vi "Read Perimeter.vi"(8 "error in (no error)":errorcluster, 11 "Circle in":refnum<class "Circle.lvclass">) -> (0 "error out":errorcluster, 2 "Perimeter":dbl, 3 "Circle out":refnum<class "Circle.lvclass">)   [LabVIEW 2015]
uses:
  Circle.lvclass
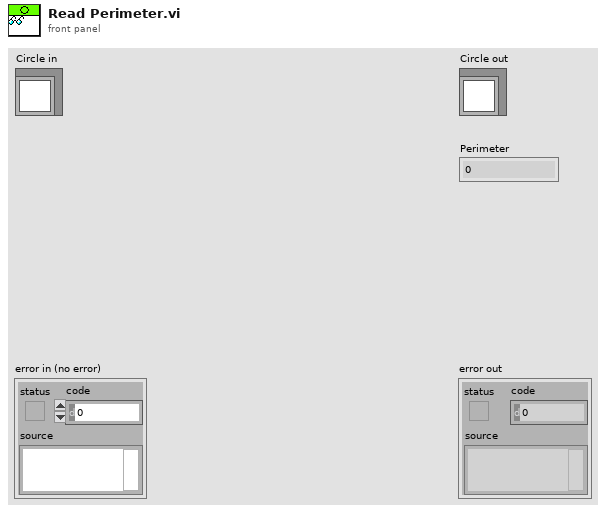
[diagram p1: front panel]
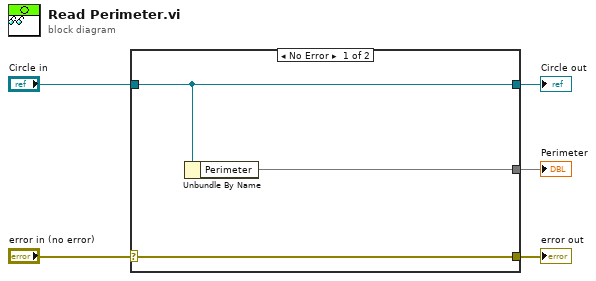
[diagram p0: block diagram]
diagram:
  n1 = case shown="No Error" "error in (no error)" {
    selector: "error in (no error)" -> [w8 w9]
    tunnel: [w8 w9] -> w4
    tunnel: [w7 w10] -> w2
    tunnel: "Circle in" -> [w7 w10]
    tunnel: [w6 _] -> w1
    frame No Error {
      n2 = Unbundle By Name(w7) -> ("Perimeter"=w6)
    }
    frame Error {
    }
  }
  "error out" <- w4
  "Circle out" <- w2
  "Perimeter" <- w1
